vi "Control Panel.vi"(8 "error in (no error)":errorcluster, 11 "Translation Stages in":refnum<class "Translation Stages.lvclass">) -> (0 "error out":errorcluster, 3 "Translation Stages out":refnum<class "Translation Stages.lvclass">)   [LabVIEW 2012, in "Translation Stages.lvclass"]
uses:
  Translation Stages.lvclass
  Global/GPIB Numbers.vi
  Utility Classes/Scannable/Scannable.lvclass
panel:
  in  "Step Rate Set":dbl=2000.0 min=32.0 max=3000.0 step=1.0
  out "Step Rate":ext
  in  "Set Step Rate":bool
  in  "Combined Position Set":dbl[unit] format="%#_8g"
  in  "Go to combined position\n(minimizing fine axis)":bool
  in  "Go to fine position":bool
  in  "Read to Control":bool
  in  "Fine Axis Set (um)":dbl[unit]
  in  "Coarse Axis Set (um)":dbl[unit]
  out "Combined Position (um)":ext[unit] format="%#_8g"
  out "Coarse Axis (um)":ext[unit]
  out "Fine Axis (um)":ext[unit]
  in  "Go to coarse position":bool
  in  "Read Positions":bool
  out "fine axis (steps)":dbl
  out "coarse axis(steps)":dbl
  in  "Calibrate Zero Positions":bool
  in  "stop":bool
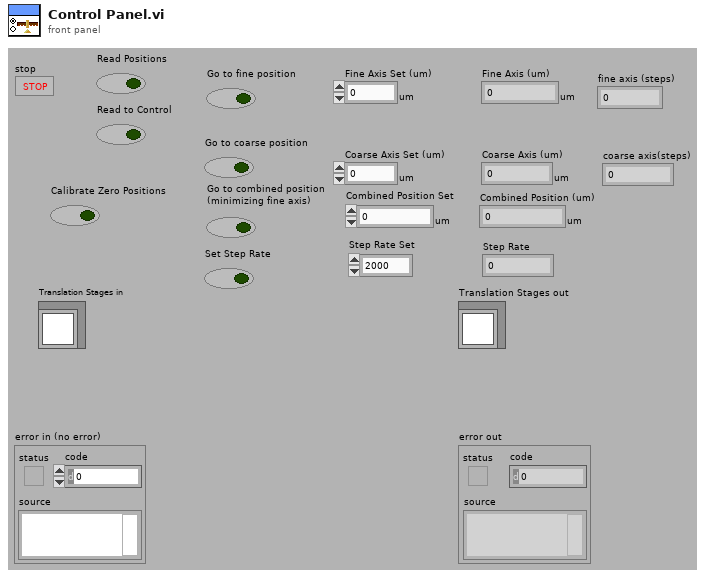
[diagram p1: front panel]
types:
  T1 = typedef "GPIB Type Def.ctl" = cluster{"Name":string, "bus":dbl, "GPIB":dbl, "GPIB as string":string, "byte":i32, "VISA Resource Name":refnum<visa-resource-name>}
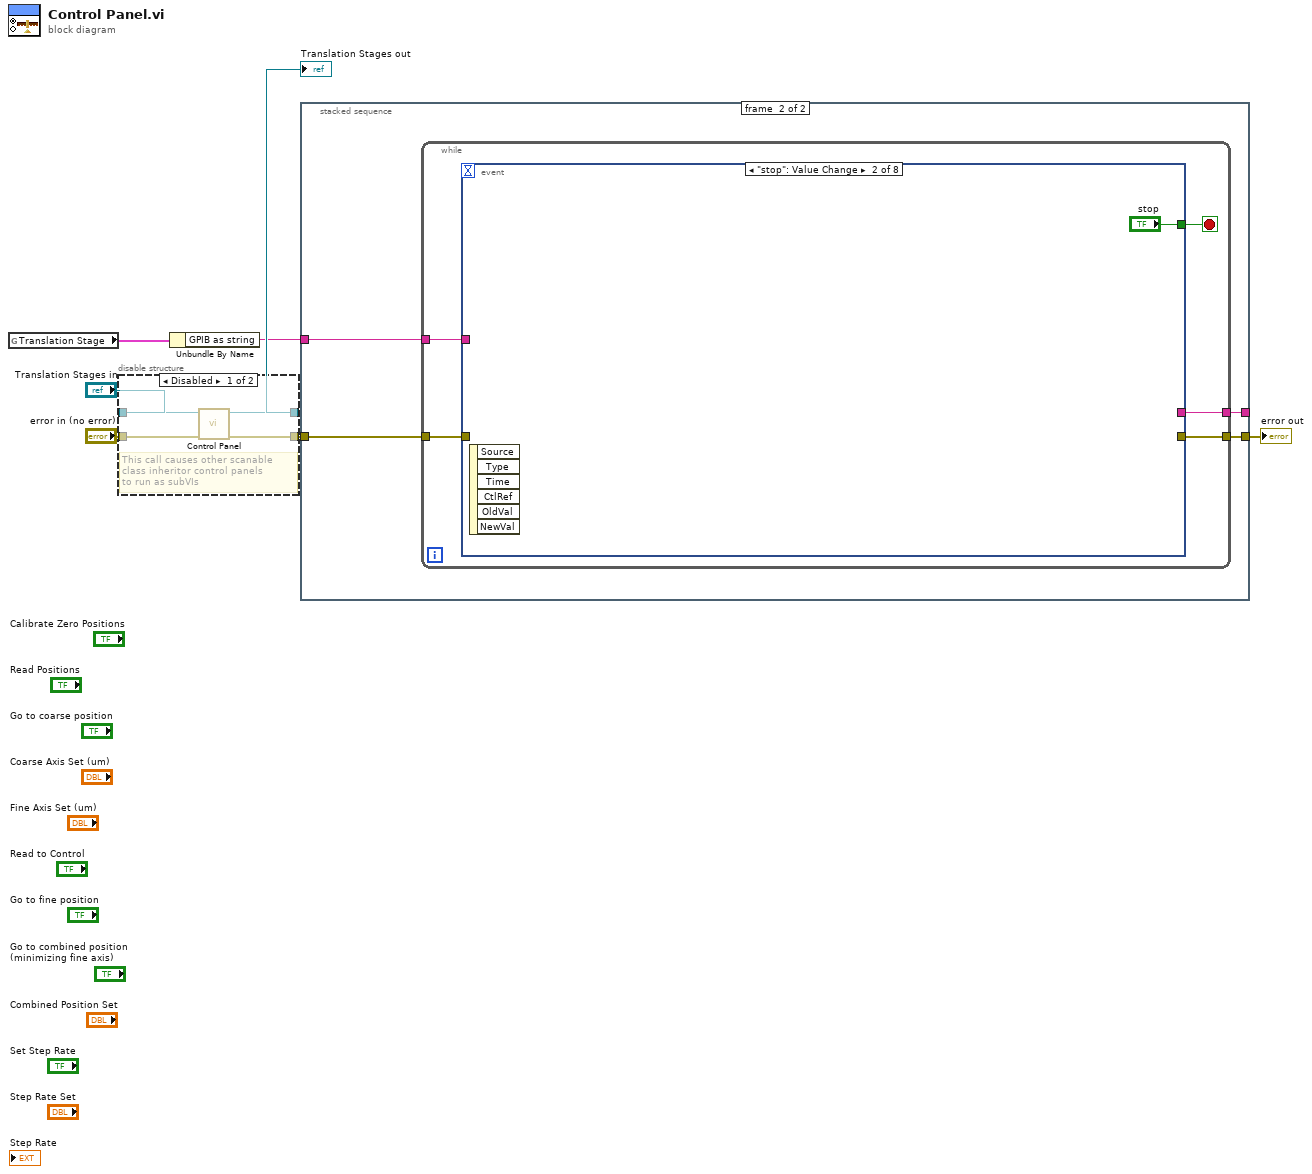
[diagram p0: block diagram]
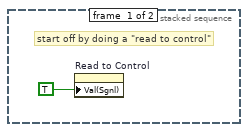
[diagram p3: hidden frame]
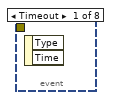
[diagram p4: hidden frame]
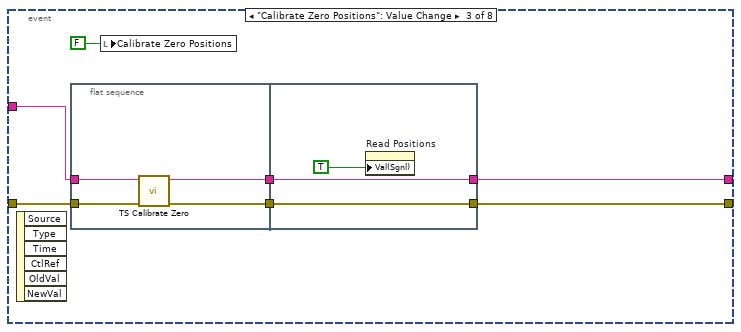
[diagram p5: hidden frame]
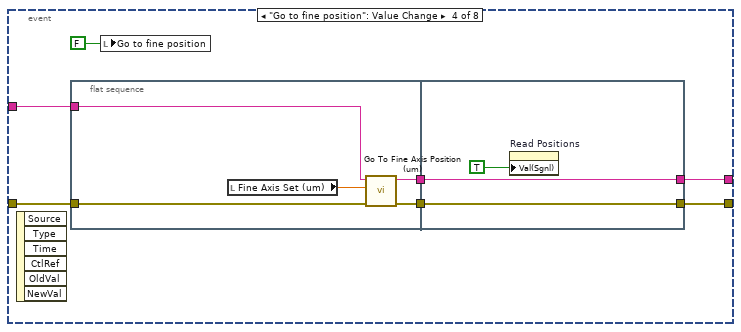
[diagram p6: hidden frame]
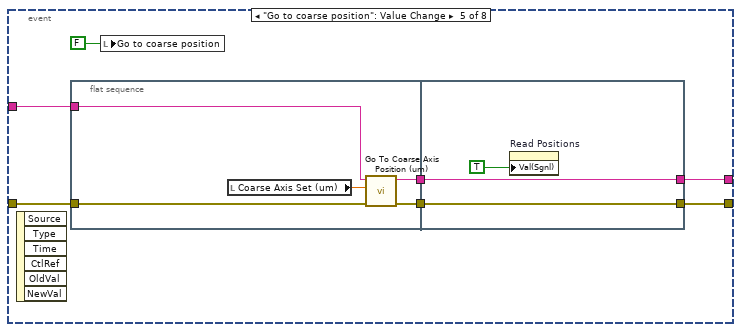
[diagram p7: hidden frame]
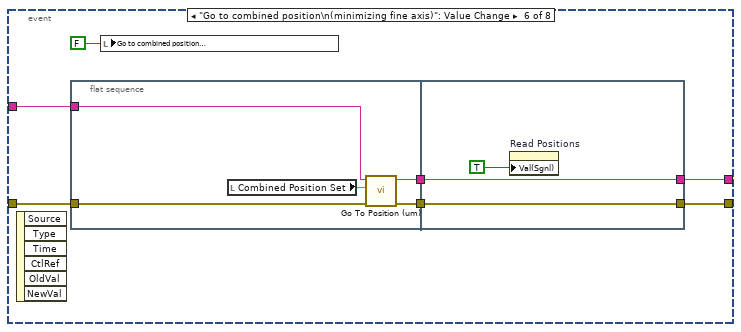
[diagram p8: hidden frame]
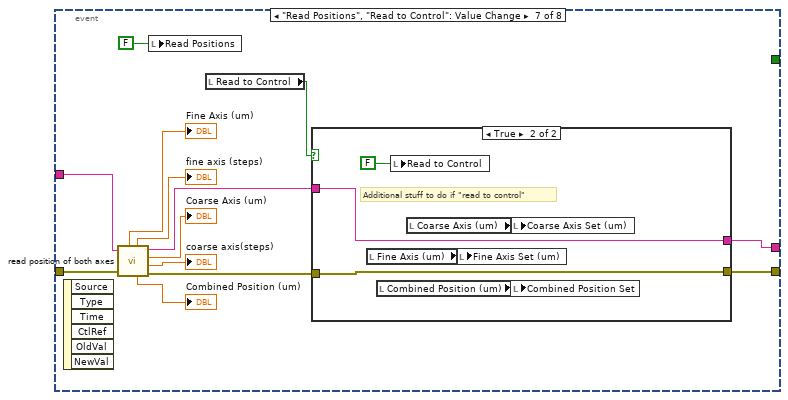
[diagram p9: hidden frame]
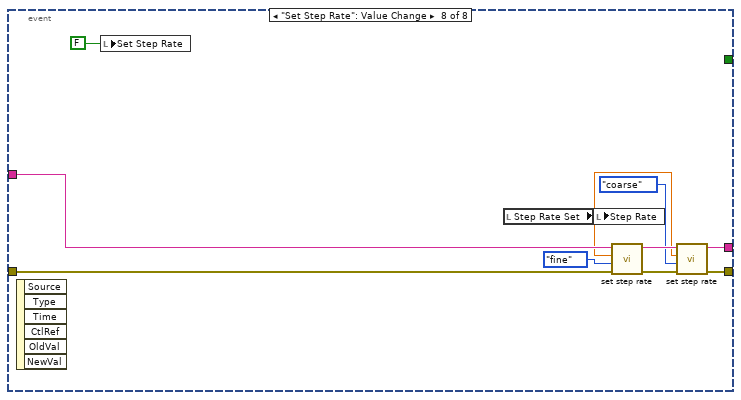
[diagram p11: hidden frame]
diagram:
  n1 = global read "GPIB Numbers.vi" "Translation Stage"() -> (w2:T1)
  n2 = disable-structure shown="Disabled" {
    disable-tunnel: [w11 w13] -> w7
    disable-tunnel: "error in (no error)" -> [w10 w12]
    disable-tunnel: "Translation Stages in" -> [w9 w13]
    disable-tunnel: [w8 w12] -> w4
    frame Disabled {
      # "This call causes other scanable\nclass inheritor control panels\nto run as subVIs"
      n3 = call-parent "Control Panel.vi"("error in (no error)"=w10, "Instrument in"=w9) -> ("error out"=w8:errorcluster, "Instrument out"=w11:refnum<class "Translation Stages.lvclass">)  [unwired: 8 out]
    }
    frame Enabled {
    }
  }
  "Translation Stages out" <- w7
  n4 = Unbundle By Name(w2) -> ("GPIB as string"=w1:string)
  n5 = stacked-sequence {
    tunnel: w4 -> [_ w18]
    tunnel: [_ w17] -> w3
    tunnel: w1 -> [_ w16]
    tunnel: [_ w15] -> _
    frame #0 {
      # "start off by doing a \"read to control\""
      n6 = property on="Read to Control" class="Bool (strict)"("Val(Sgnl)"=TRUE ("Value (Signaling)")) -> ()  [unwired: 2 in, 2 out]
    }
    frame #1 {
      n7 = while {
        tunnel: w18 -> [w22]
        tunnel: [w21] -> w17
        tunnel: w16 -> [w20]
        tunnel: [w19] -> w15
        stop <- w23 stop-if-true
        n8 = event shown="[1] \"stop\": Value Change" {
          selector: _ -> [_ _ _ _ _ _ _ _]
          dyn-events: _ -> [_ _ _ _ _ _ _ _]
          timeout: _ -> [_ _ _ _ _ _ _ _]
          tunnel: [_ "stop" _ _ _ _ _ _] -> w23
          tunnel: w22 -> [_ _ w27 w42 w57 w72 w95 w113]
          tunnel: [_ _ w30 w44 w58 w73 w89 w107] -> w21
          tunnel: w20 -> [_ _ w28 w41 w54 w71 w88 w114]
          tunnel: [_ _ w29 w39 w56 w69 w84 w108] -> w19
          event Timeout {
            n9 = event-data() -> ()  [unwired: 3 out]
          }
          event "stop": Value Change {
            n10 = event-data() -> ()  [unwired: 7 out]
          }
          event "Calibrate Zero Positions": Value Change {
            n11 = event-data() -> ()  [unwired: 7 out]
            n12 = flat-sequence {
              tunnel: w28 -> [w35]
              tunnel: w27 -> [w34]
              tunnel: [w33] -> w26
              tunnel: [w32] -> w25
              tunnel: [w36] -> w30
              tunnel: [w37] -> w29
              tunnel: w26 -> [w37]
              tunnel: w25 -> [w36]
              frame #0 {
                n13 = call "TS Calibrate Zero.vi"("error out"=w34, "GPIB as string"=w35) -> ("error out 2"=w32:errorcluster, "GPIB # (out)"=w33:string)  [unwired: 8 out]
              }
              frame #1 {
                n14 = property on="Read Positions" class="Bool (strict)"("Val(Sgnl)"=TRUE ("Value (Signaling)")) -> ()  [unwired: 2 in, 2 out]
              }
            }
            n15 = local write "Calibrate Zero Positions"(FALSE ("Calibrate Zero Position")) -> ()
          }
          event "Go to fine position": Value Change {
            n16 = event-data() -> ()  [unwired: 7 out]
            n17 = flat-sequence {
              tunnel: [w49] -> w43
              tunnel: w42 -> [w48]
              tunnel: w41 -> [w47]
              tunnel: [w46] -> w40
              tunnel: [w52] -> w44
              tunnel: w43 -> [w52]
              tunnel: w40 -> [w51]
              tunnel: [w51] -> w39
              frame #0 {
                n18 = local read "Fine Axis Set (um)"() -> (w50:dbl[unit])
                n19 = call "Go To Fine Axis Position (um).vi"("error in"=w48, "Fine Axis Position (um)"=w50, "GPIB # (in): def. 6"=w47) -> ("error out"=w49:errorcluster, "GPIB # (out)"=w46:string)  [unwired: 7 out]
              }
              frame #1 {
                n20 = property on="Read Positions" class="Bool (strict)"("Val(Sgnl)"=TRUE ("Value (Signaling)")) -> ()  [unwired: 2 in, 2 out]
              }
            }
            n21 = local write "Go to fine position"(FALSE ("Go to fine position")) -> ()
          }
          event "Go to coarse position": Value Change {
            n22 = event-data() -> ()  [unwired: 7 out]
            n23 = flat-sequence {
              tunnel: [w63] -> w60
              tunnel: w57 -> [w64]
              tunnel: [w62] -> w55
              tunnel: w54 -> [w61]
              tunnel: [w67] -> w58
              tunnel: w60 -> [w67]
              tunnel: [w66] -> w56
              tunnel: w55 -> [w66]
              frame #0 {
                n24 = local read "Coarse Axis Set (um)"() -> (w65:dbl[unit])
                n25 = call "Go To Coarse Axis Position (um).vi"("error in (no error)"=w64, "Coarse Axis Position (um)"=w65, "GPIB # (in): def. 6"=w61) -> ("error out"=w63:errorcluster, "GPIB # (out)"=w62:string)  [unwired: 7 out]
              }
              frame #1 {
                n26 = property on="Read Positions" class="Bool (strict)"("Val(Sgnl)"=TRUE ("Value (Signaling)")) -> ()  [unwired: 2 in, 2 out]
              }
            }
            n27 = local write "Go to coarse position"(FALSE ("Go to fine position")) -> ()
          }
          event "Go to combined position\n(minimizing fine axis)": Value Change {
            n28 = event-data() -> ()  [unwired: 7 out]
            n29 = flat-sequence {
              tunnel: [w78] -> w75
              tunnel: w72 -> [w79]
              tunnel: w71 -> [w77]
              tunnel: [w76] -> w70
              tunnel: [w82] -> w73
              tunnel: w75 -> [w82]
              tunnel: [w81] -> w69
              tunnel: w70 -> [w81]
              frame #0 {
                n30 = local read "Combined Position Set"() -> (w80:dbl[unit])
                n31 = call "Go To Position (um).vi"("error in (no error)"=w79, "Position (um)"=w80, "GPIB # (in): def. 6"=w77) -> ("error out"=w78:errorcluster, "GPIB # (out)"=w76:string)  [unwired: 7 out]
              }
              frame #1 {
                n32 = property on="Read Positions" class="Bool (strict)"("Val(Sgnl)"=TRUE ("Value (Signaling)")) -> ()  [unwired: 2 in, 2 out]
              }
            }
            n33 = local write "Go to combined position\n(minimizing fine axis)"(FALSE ("Go to fine position")) -> ()
          }
          event "Read Positions", "Read to Control": Value Change {
            n34 = event-data() -> ()  [unwired: 7 out]
            n35 = call "read position of both axes.vi"("GPIB # (in): def. 6"=w88, "error in (no error)"=w95) -> ("fine axis (um)"=→"Fine Axis (um)":ext[unit], "fine axis (steps)"=→"fine axis (steps)":dbl, "GPIB # (out)"=w85:string, "coarse axis (um)"=→"Coarse Axis (um)":ext[unit], "combined position (um)"=→"Combined Position (um)":ext[unit], "coarse axis(steps)"=→"coarse axis(steps)":dbl, "error out"=w90:errorcluster)  [unwired: 2 out]
            n36 = local write "Read Positions"(FALSE ("Read Positions")) -> ()
            n37 = local read "Read to Control"() -> (w91:bool)
            n38 = case shown="True" w91 {
              tunnel: w90 -> [w98 w100]
              tunnel: [w98 w100] -> w89
              tunnel: w85 -> [w97 w99]
              tunnel: [w97 w99] -> w84
              frame False {
              }
              frame True {
                # "Additional stuff to do if \"read to control\""
                n39 = local read "Fine Axis (um)"() -> (w102:ext[unit])
                n40 = local read "Combined Position (um)"() -> (w101:ext[unit])
                n41 = local write "Read to Control"(FALSE ("Read Positions")) -> ()
                n42 = local read "Coarse Axis (um)"() -> (w103:ext[unit])
                n43 = local write "Fine Axis Set (um)"(w102) -> ()
                n44 = local write "Coarse Axis Set (um)"(w103) -> ()
                n45 = local write "Combined Position Set"(w101) -> ()
              }
            }
          }
          event "Set Step Rate": Value Change {
            n46 = event-data() -> ()  [unwired: 7 out]
            n47 = local write "Set Step Rate"(FALSE) -> ()
            n48 = local read "Step Rate Set"() -> (w105:dbl)
            n49 = local write "Step Rate"(w105) -> ()
            n50 = call "set step rate.vi"("error in"=w113, "axis (def: fine)"=enum16{"fine", "coarse"}."fine", "step rate"=w105, "GPIB # (in): def. 6"=w114) -> ("error out"=w110:errorcluster, "GPIB # (out)"=w111:string)  [unwired: 6 out]
            n51 = call "set step rate.vi"("error in"=w110, "axis (def: fine)"=enum16{"fine", "coarse"}."coarse", "step rate"=w105, "GPIB # (in): def. 6"=w111) -> ("error out"=w107:errorcluster, "GPIB # (out)"=w108:string)  [unwired: 6 out]
          }
        }
      }
    }
  }
  "error out" <- w3
